vi "generate_y galvo_voltages.vi"(5 "xy view?":bool, 6 "x galvo":i16, 7 "focus mode?":bool, 8 "derived values":T1, 9 "scan specification":T4={"x amplitude"=0, "x resolution (pixels)"=0, "x offset fly-forward (iterations)"=0, "x offset fly-back (iterations)"=0, "y resolution (nr. of lines)"=0, "y step size"=0, "iterations per pixel"=0, "number of frames"=0, "y offset (pixels)"=0, "number of y-brake lines  (before y-fly-back)"=0, "number y-brake lines (after y-fly-back)"=0, "number of y-fly-back steps"=8, "lines per z step"=0, "number of z/intensity tuples"=0, "number of repetitions (volumes or planes)"=0, "z step size derived"=0, "choose the beginning of z scan"=FALSE, "number of frames (settings)"=0, "FPGA trajectory?"=FALSE, "Pockels cell voltage (bits)"=0, "Vy min(bits)"=0, "Vz min(bits)"=0}, 10 "counter cluster in":T2, 11 "resonant trigger":bool) -> (0 "acquire?":bool, 1 "fly-back acquisition phase?":bool, 2 "counter cluster out":T2, 3 "DAC voltages":T3 {"ch6" max=4095 step=1; "ch5" max=4095 step=1; "ch4" max=4095 step=1; "ch3" max=4095 step=1; "ch2" max=4095 step=1; "ch1" max=4095 step=1; "ch0" max=4095 step=1}, 4 "calculate COM at the end of volume?":bool)   [LabVIEW 2010]
uses:
  scan_specification_cluster.ctl
  common_typedefs/DAC_voltage_cluster.ctl
  counter_cluster.ctl
  derived_values_cluster.ctl
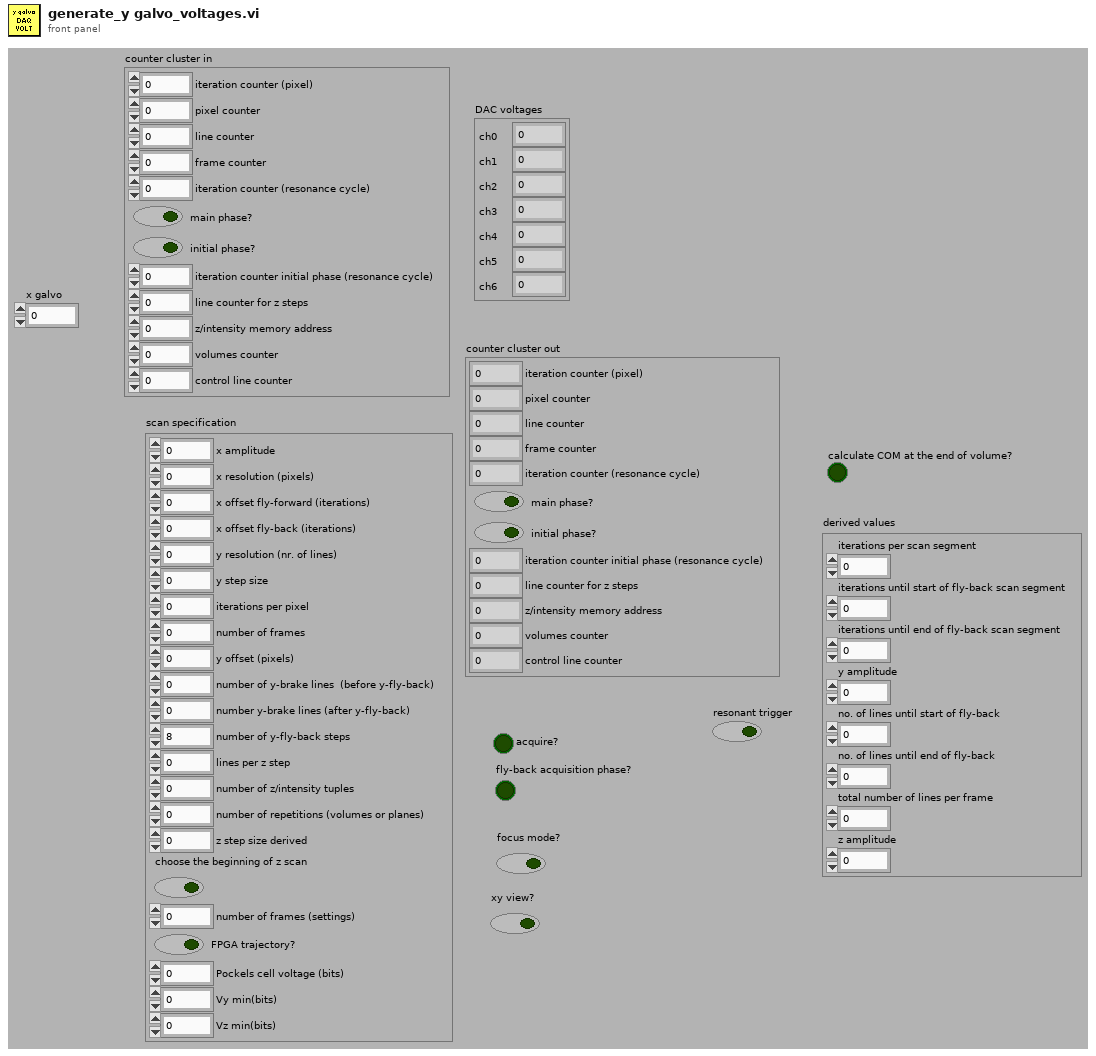
[diagram p1: front panel]
types:
  T1 = typedef "derived_values_cluster.ctl" = cluster{"iterations per scan segment":u16, "iterations until start of fly-back scan segment":u16, "iterations until end of fly-back scan segment":u16, "y amplitude":u16, "no. of lines until start of fly-back":u16, "no. of lines until end of fly-back":u16, "total number of lines per frame ":u16, "z amplitude":u16}
  T2 = typedef "counter_cluster.ctl" = cluster{"iteration counter (pixel)":u16, "pixel counter":u16, "line counter":u16, "frame counter":u16, "iteration counter (resonance cycle)":u16, "main phase?":bool, "initial phase?":bool, "iteration counter initial phase (resonance cycle)":u16, "line counter for z steps":u16, "z/intensity memory address":u32, "volumes counter":u16, "control line counter":u16}
  T3 = typedef "DAC_voltage_cluster.ctl" = cluster{"ch0":u16, "ch1":i16, "ch2":i16, "ch3":i16, "ch4":u16, "ch5":u16, "ch6":u16}
  T4 = typedef "scan_specification_cluster.ctl" = cluster{"x amplitude":u16, "x resolution (pixels)":u16, "x offset fly-forward (iterations)":u16, "x offset fly-back (iterations)":u16, "y resolution (nr. of lines)":u16, "y step size":u16, "iterations per pixel":u16, "number of frames":i32, "y offset (pixels)":u16, "number of y-brake lines  (before y-fly-back)":u16, "number y-brake lines (after y-fly-back)":u16, "number of y-fly-back steps":u16, "lines per z step":u16, "number of z/intensity tuples":u16, "number of repetitions (volumes or planes)":i32, "z step size derived":u16, "choose the beginning of z scan":bool, "number of frames (settings)":i32, "FPGA trajectory?":bool, "Pockels cell voltage (bits)":i16, "Vy min(bits)":i16, "Vz min(bits)":i16}
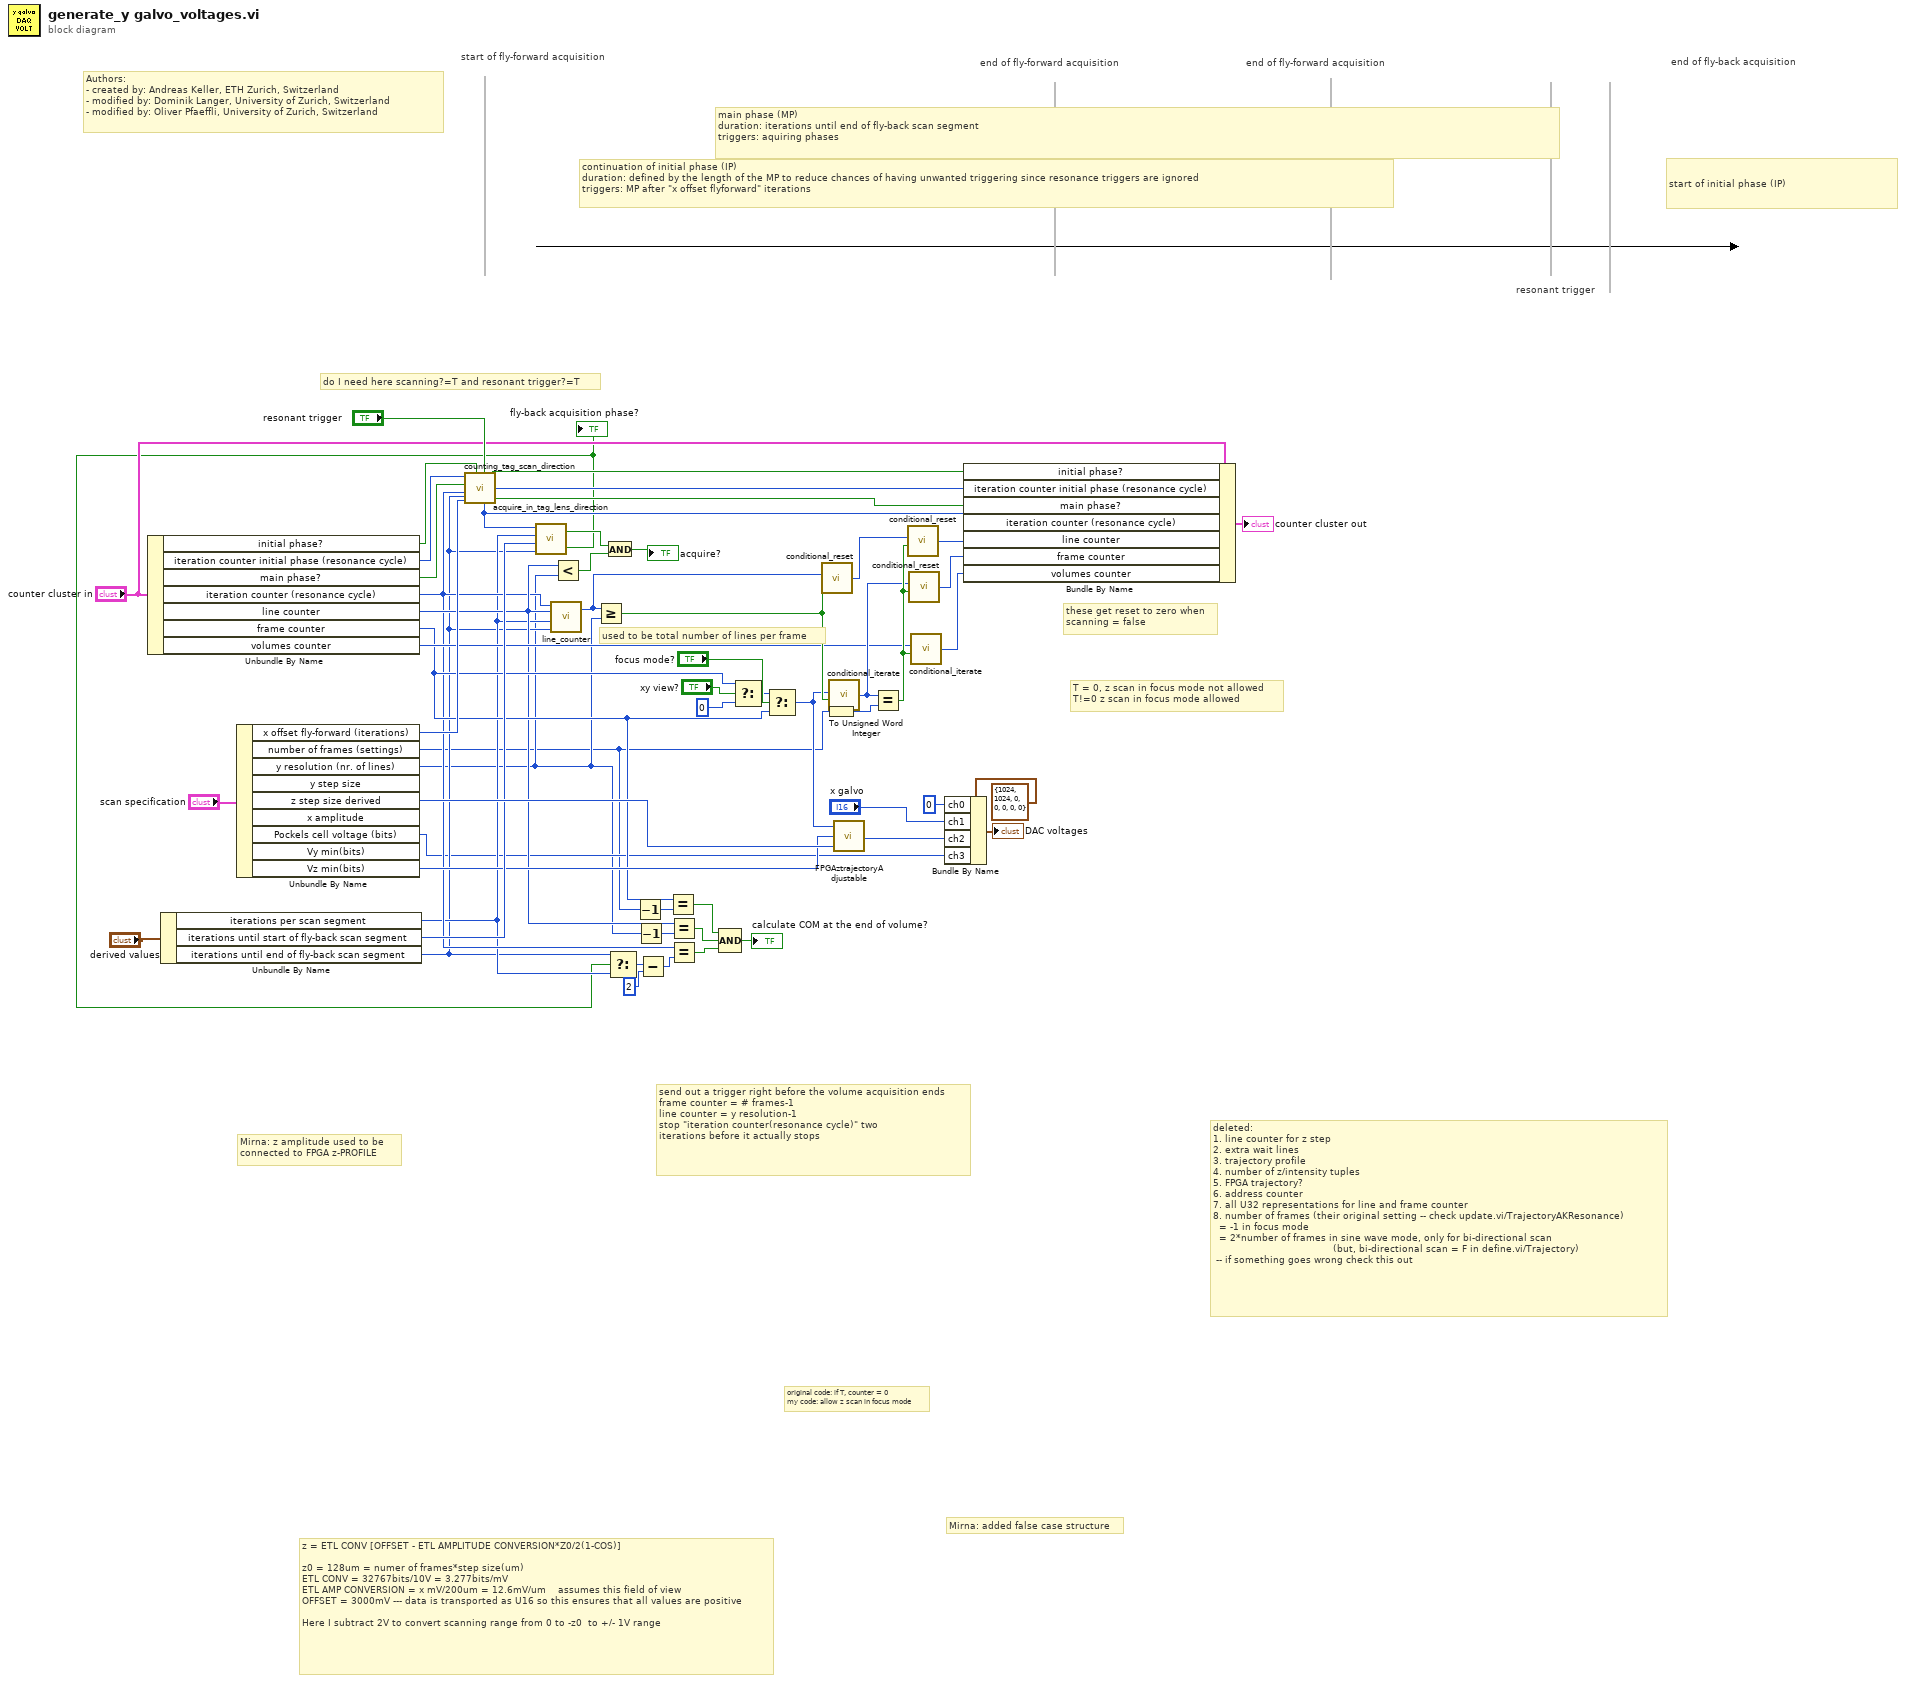
[diagram p0: block diagram]
diagram:
  # "do I need here scanning?=T and resonant trigger?=T"
  # "these get reset to zero when \nscanning = false"
  # "used to be total number of lines per frame"
  # "send out a trigger right before the volume acquisition ends\nframe counter = # frames-1\nline counter = y resolution-1\nstop \"iteration counter(resonance cycle)\" two\niterations before it actually stops"
  # "Mirna: z amplitude used to be \nconnected to FPGA z-PROFILE"
  # "T = 0, z scan in focus mode not allowed\nT!=0 z scan in focus mode allowed"
  # "deleted: \n1. line counter for z step\n2. extra wait lines\n3. trajectory profile\n4. number of z/intensity tuples\n5. FPGA trajectory?\n6. address counter\n7. all U32 representations for line and frame counter\n8. number of frames (their original setting -- check update.vi/TrajectoryAKResonance)\n  = -1 in focus mode \n  = 2*number of frames in sine wave mode, only for bi-directional scan\n                                        (but, bi-directional scan = F in define.vi/Trajectory)\n -- if something goes wrong check this out"
  # "z = ETL CONV [OFFSET - ETL AMPLITUDE CONVERSION*Z0/2(1-COS)]\n\nz0 = 128um = numer of frames*step size(um)\nETL CONV = 32767bits/10V = 3.277bits/mV\nETL AMP CONVERSION = x mV/200um = 12.6mV/um    assumes this field of view\nOFFSET = 3000mV --- data is transported as U16 so this ensures that all values are positive\n\nHere I subtract 2V to convert scanning range from 0 to -z0  to +/- 1V range"
  # "original code: if T, counter = 0\nmy code: allow z scan in focus mode"
  # "Mirna: added false case structure"
  # "start of initial phase (IP)"
  # "continuation of initial phase (IP)\nduration: defined by the length of the MP to reduce chances of having unwanted triggering since resonance triggers are ignored\ntriggers: MP after \"x offset flyforward\" iterations"
  # "end of fly-back acquisition"
  # "end of fly-forward acquisition"
  # "end of fly-forward acquisition"
  # "start of fly-forward acquisition"
  # "main phase (MP)\nduration: iterations until end of fly-back scan segment\ntriggers: aquiring phases"
  # "resonant trigger"
  # "Authors: \n- created by: Andreas Keller, ETH Zurich, Switzerland\n- modified by: Dominik Langer, University of Zurich, Switzerland\n- modified by: Oliver Pfaeffli, University of Zurich, Switzerland"
  n1 = Unbundle By Name("counter cluster in") -> ("initial phase?"=w52:bool, "iteration counter initial phase (resonance cycle)"=w43:u16, "main phase?"=w49:bool, "iteration counter (resonance cycle)"=w17:u16, "line counter"=w20:u16, "frame counter"=w26:u16, "volumes counter"=w27:u16)
  n2 = Unbundle By Name("derived values") -> ("iterations per scan segment"=w16:u16, "iterations until start of fly-back scan segment"=w42:u16, "iterations until end of fly-back scan segment"=w15:u16)
  n3 = Unbundle By Name("scan specification") -> ("x offset fly-forward (iterations)"=w41:u16, "number of frames (settings)"=w2:i32, "y resolution (nr. of lines)"=w4:u16, "z step size derived"=w47:u16, "Pockels cell voltage (bits)"=w5:i16, "Vz min(bits)"=w28:i16)  [unwired: 3 out]
  n4 = call "counting_tag_scan_direction.vi"("resonant trigger"="resonant trigger", "initial phase?"=w52, "iteration counter initial phase (resonance cycle)"=w43, "main phase?"=w49, "iterations until end of fly-back scan segment"=w15, "iteration counter (resonance cycle)"=w17, "x offset fly-forward (iterations)"=w41) -> ("initial phase? OUT"=w45:bool, "iteration counter initial phase (resonance cycle) out"=w44:u16, "main phase? OUT"=w40:bool, "iteration counter (resonance cycle) out"=w39:u16)
  n5 = call "acquire_in_tag_lens_direction.vi"("iterations until end of fly-back scan segment"=w15, "iterations until start of fly-back scan segment"=w42, "iterations per scan segment"=w16, "iteration counter (resonance cycle) out"=w39) -> ("flyback phase?"=w3:bool, "acquire during flyforward or flyback phase?"=w53:bool)
  "fly-back acquisition phase?" <- w3
  n6 = call "line_counter.vi"("iterations until end of fly-back scan segment"=w15, "iterations per scan segment"=w16, "line counter in"=w20, "iteration counter (resonance cycle)"=w17) -> ("line counter out"=w34:u16)  [unwired: 1 out]
  n7 = Less?(x=w20, y=w4) -> (x < y?=w11:bool)
  n8 = Greater Or Equal?(x=w34, y=w4) -> (x >= y?=w35:bool)
  n9 = And(x=w53, y=w11) -> (x .and. y?=→"acquire?":bool)
  n10 = Select(t=w15, s=w3, f=w16) -> (s? t:f=w14:u16)
  n11 = Decrement(x=w2) -> (x-1=w25:i32)
  n12 = Decrement(x=w4) -> (x-1=w21:u16)
  n13 = Subtract(x=w14, y=u16 2) -> (x-y=w12:u16)
  n14 = Equal?(x=w26, y=w25) -> (x = y?=w24:bool)
  n15 = Equal?(x=w20, y=w21) -> (x = y?=w19:bool)
  n16 = Equal?(x=w17, y=w12) -> (x = y?=w18:bool)
  n17 = Compound Arithmetic op=AND(w24, w19, w18) -> (→"calculate COM at the end of volume?":bool)
  n18 = Select(t=w26, s="xy view?", f=u16 0) -> (s? t:f=w29:u16)
  n19 = Select(t=w29, s="focus mode?", f=w26) -> (s? t:f=w6:u16)
  n20 = call "conditional_reset.vi"("reset?"=w35, "number in"=w34) -> ("number out"=w37:u16)  [unwired: 4 in]
  n21 = To Unsigned Word Integer(number=w2) -> (unsigned 16bit integer=w7:u16)
  n22 = call "conditional_iterate.vi"("iterate?"=w35, "number in"=w6) -> ("number out"=w33:u16)  [unwired: 4 in]
  n23 = call "FPGAztrajectoryAdjustable.vi"("z step size derived"=w47, "Vz min (bits)"=w28, "z/intensity memory address"=w6) -> ("Z trajectory"=w48:i16)
  n24 = Equal?(x=w33, y=w7) -> (x = y?=w38:bool)
  n25 = call "conditional_reset.vi"("reset?"=w38, "number in"=w37) -> ("number out"=w50:u16)  [unwired: 4 in]
  n26 = call "conditional_reset.vi"("reset?"=w38, "number in"=w33) -> ("number out"=w36:u16)  [unwired: 4 in]
  n27 = call "conditional_iterate.vi"("iterate?"=w38, "number in"=w27) -> ("number out"=w51:u16)  [unwired: 4 in]
  n28 = Bundle By Name(cluster=T3 {"ch0"=1024, "ch1"=1024, "ch2"=0, "ch3"=0, "ch4"=0, "ch5"=0, "ch6"=0} ("DAC voltage"), "ch0"=u16 0, "ch1"="x galvo", "ch2"=w48, "ch3"=w5) -> (→"DAC voltages":T3)
  n29 = Bundle By Name(cluster="counter cluster in", "initial phase?"=w45, "iteration counter initial phase (resonance cycle)"=w44, "main phase?"=w40, "iteration counter (resonance cycle)"=w39, "line counter"=w50, "frame counter"=w36, "volumes counter"=w51) -> (→"counter cluster out":T2)
